vi "Configure Real Time Eye.vi"(0 "VISA resource name":refnum<visa-resource-name>, 1 "Waveform Source (0: Channel 1)":i32(ring) items=["Channel 1", "Channel 2", "Channel 3", "Channel 4", "Common 1", "Common 2", "Differential 1", "Differential 2", "Memory 1", "Memory 2", "Memory 3", "Memory 4", "Function 1", "Function 2", "Function 3", "Function 4", "Function 5", "Function 6", "Function 7", "Function 8", "Function 9", "Function 10", "Function 11", "Function 12", "Function 13", "Function 14", "Function 15", "Function 16"], 5 "Enable Real Time Eye (T: Enable)":bool=TRUE, 7 "Data Bits (0: Both)":i32(ring) items=["Both", "Deemphasis", "Transition", "Pattern"], 9 "Bit Pattern":string, 11 "error in (no error)":errorcluster, 12 "Bit Cursor (0: Bit 0)":u16(ring) items=["Bit 0", "Bit 1", "Bit 2", "Bit 3", "Bit 4", "Bit 5", "Bit 6", "Bit 7"]) -> (4 "VISA resource name out":refnum<visa-resource-name>, 15 "error out":errorcluster)   [LabVIEW 2013, in "Agilent 90000 Series.lvlib"]
doc: "Configures the real time eye parameters."
uses:
  Agilent 90000 Series.lvlib
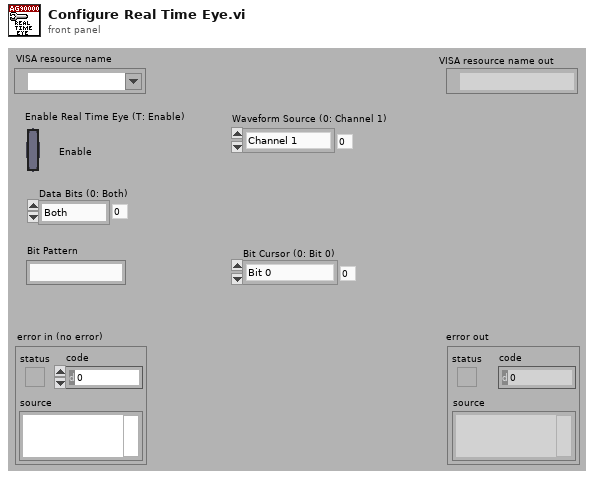
[diagram p1: front panel]
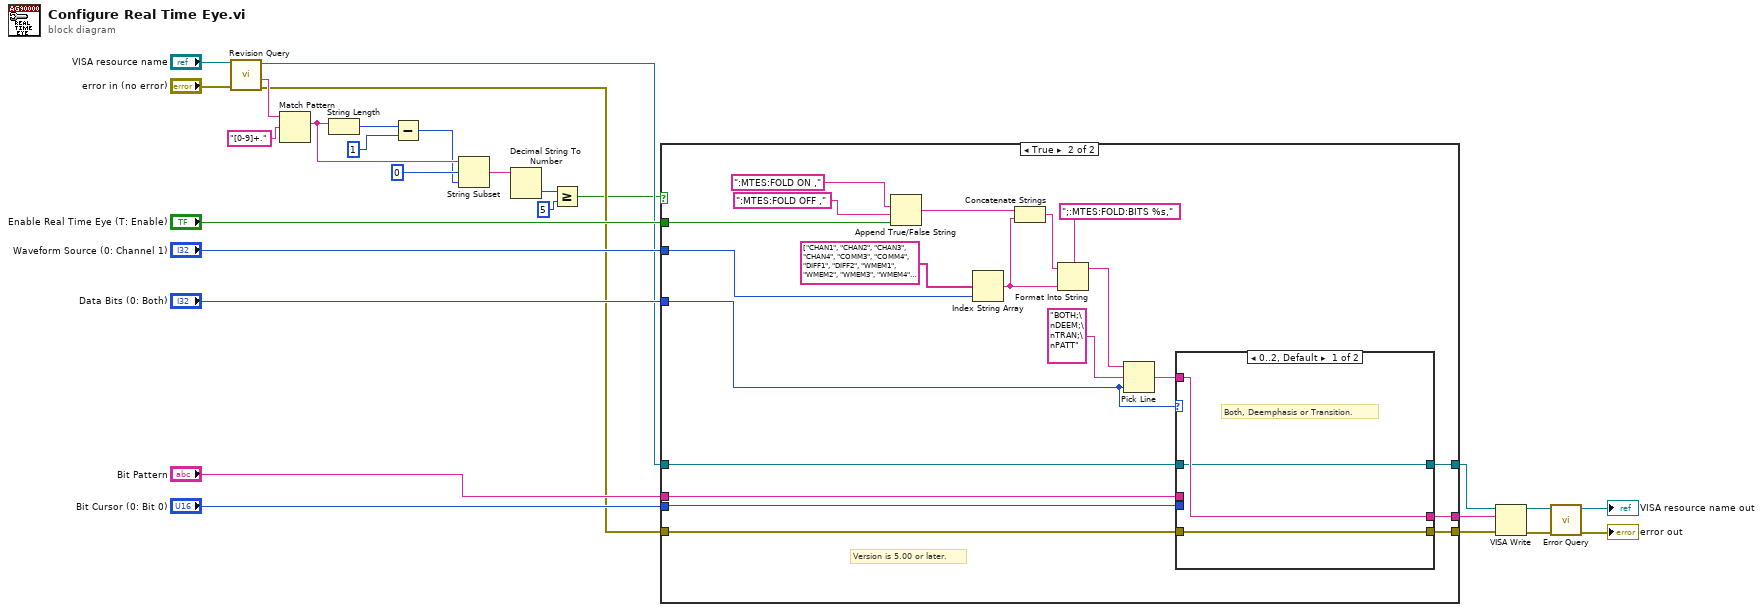
[diagram p0: block diagram]
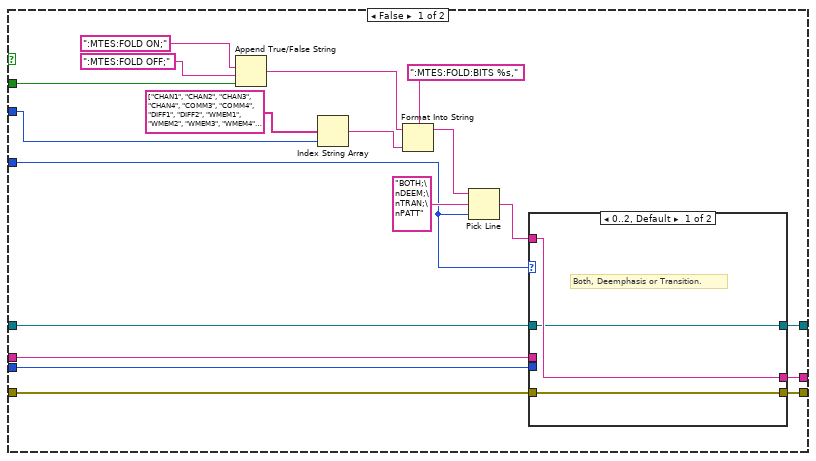
[diagram p2: hidden frame]
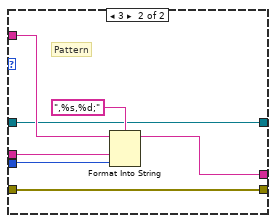
[diagram p3: hidden frame]
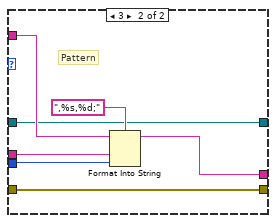
[diagram p4: hidden frame]
diagram:
  n1 = call "Revision Query.vi"("error in (no error)"="error in (no error)", "VISA resource name"="VISA resource name") -> ("error out"=w5:errorcluster, "Instrument Firmware Revision"=w9:string, "VISA resource name out"=w6:refnum<visa-resource-name>)  [unwired: 6 in, 1 out]
  n2 = Match Pattern(string=w9, regular expression="[0-9]+.") -> (match substring=w16:string)  [unwired: 1 in, 3 out]
  n3 = String Length(string=w16) -> (length=w14:i32)
  n4 = Subtract(x=w14, y=1) -> (x-y=w12:i32)
  n5 = String Subset(string=w16, offset (0)=0, length (rest)=w12) -> (substring=w11:string)
  n6 = Decimal String To Number(string=w11) -> (number=w10:i32)  [unwired: 2 in, 1 out]
  n7 = Greater Or Equal?(x=w10, y=5) -> (x >= y?=w1:bool)
  n8 = case shown="True" w1 {
    tunnel: "Enable Real Time Eye (T: Enable)" -> [w39 w74]
    tunnel: [w30 w68] -> w22
    tunnel: [w29 w66] -> w3
    tunnel: w5 -> [w34 w67]
    tunnel: w6 -> [w35 w65]
    tunnel: [w31 w64] -> w4
    tunnel: "Waveform Source (0: Channel 1)" -> [w37 w73]
    tunnel: "Data Bits (0: Both)" -> [w28 w57]
    tunnel: "Bit Pattern" -> [w33 w70]
    tunnel: "Bit Cursor (0: Bit 0)" -> [w32 w69]
    frame False {
      n9 = Append True/False String(1:w39, 2:":MTES:FOLD OFF;" ("false string"), 3:":MTES:FOLD ON;" ("true string")) -> (0:w38:string)  [unwired: 1 out]
      n10 = Index String Array(1:w37, 2:string[] ["CHAN1", "CHAN2", "CHAN3", "CHAN4", "COMM3", "COMM4", "DIFF1", "DIFF2", "WMEM1", "WMEM2", "WMEM3", "WMEM4", "FUNC1", "FUNC2", "FUNC3", "FUNC4", "FUNC5", "FUNC6", "FUNC7", "FUNC8", "FUNC9", "FUNC10", "FUNC11", "FUNC12", "FUNC13", "FUNC14", "FUNC15", "FUNC16"] ("string array")) -> (0:w41:string)  [unwired: 1 in]
      n11 = Format Into String(format string=":MTES:FOLD:BITS %s," ("string (\"\")"), initial string=w38, w41) -> (resulting string=w40:string)  [unwired: 1 in, 1 out]
      n12 = Pick Line(string ("")=w40, multi-line string="BOTH;\nDEEM;\nTRAN;\nPATT", line index=w28) -> (output string=w36:string)
      n13 = case shown="0..2, Default" w28 {
        tunnel: [w49 w52] -> w30
        tunnel: w36 -> [w49 w53]
        tunnel: w33 -> [_ w55]
        tunnel: w32 -> [_ w54]
        tunnel: w34 -> [w48 w51]
        tunnel: [w48 w51] -> w29
        tunnel: w35 -> [w47 w50]
        tunnel: [w47 w50] -> w31
        frame 0..2, Default {
          # "Both, Deemphasis or Transition."
        }
        frame 3 {
          # "Pattern"
          n14 = Format Into String(format string=",%s,%d;", initial string=w53, w55, w54) -> (resulting string=w52:string)  [unwired: 1 in, 1 out]
        }
      }
    }
    frame True {
      # "Version is 5.00 or later."
      n15 = Append True/False String(1:w74, 2:":MTES:FOLD OFF ," ("false string"), 3:":MTES:FOLD ON ," ("true string")) -> (0:w61:string)  [unwired: 1 out]
      n16 = Index String Array(1:w73, 2:string[] ["CHAN1", "CHAN2", "CHAN3", "CHAN4", "COMM3", "COMM4", "DIFF1", "DIFF2", "WMEM1", "WMEM2", "WMEM3", "WMEM4", "FUNC1", "FUNC2", "FUNC3", "FUNC4", "FUNC5", "FUNC6", "FUNC7", "FUNC8", "FUNC9", "FUNC10", "FUNC11", "FUNC12", "FUNC13", "FUNC14", "FUNC15", "FUNC16"] ("string array")) -> (0:w59:string)  [unwired: 1 in]
      n17 = Concatenate Strings(w61, w59) -> (w60:string)
      n18 = Format Into String(format string=";:MTES:FOLD:BITS %s," ("string (\"\")"), initial string=w60, w59) -> (resulting string=w58:string)  [unwired: 1 in, 1 out]
      n19 = Pick Line(string ("")=w58, multi-line string="BOTH;\nDEEM;\nTRAN;\nPATT", line index=w57) -> (output string=w71:string)
      n20 = case shown="0..2, Default" w57 {
        tunnel: [w79 w82] -> w68
        tunnel: w71 -> [w79 w83]
        tunnel: w70 -> [_ w85]
        tunnel: w69 -> [_ w84]
        tunnel: w67 -> [w78 w81]
        tunnel: [w78 w81] -> w66
        tunnel: w65 -> [w77 w80]
        tunnel: [w77 w80] -> w64
        frame 0..2, Default {
          # "Both, Deemphasis or Transition."
        }
        frame 3 {
          # "Pattern"
          n21 = Format Into String(format string=",%s,%d;", initial string=w83, w85, w84) -> (resulting string=w82:string)  [unwired: 1 in, 1 out]
        }
      }
    }
  }
  n22 = VISA Write(VISA resource name=w4, write buffer=w22, error in (no error)=w3) -> (VISA resource name out=w27:refnum<visa-resource-name>, error out=w26:errorcluster)  [unwired: 1 out]
  n23 = call "Error Query.vi"("error in (no error)"=w26, "VISA resource name"=w27) -> ("error out"=→"error out":errorcluster, "VISA resource name out"=→"VISA resource name out":refnum<visa-resource-name>)  [unwired: 8 out]
